vi "mul.vi"(11 "arguments":T1[](array[typedef])) -> (3 "Expression":T1)   [LabVIEW 2020]
uses:
  ExpressionType.ctl
  Expression.ctl
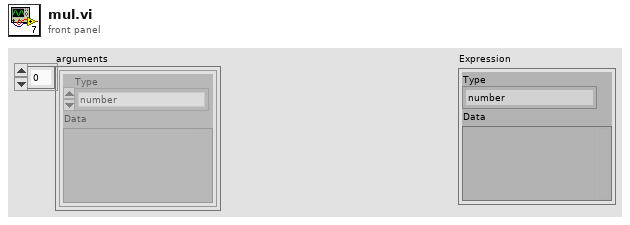
[diagram p1: front panel]
types:
  T1 = typedef "Expression.ctl" = cluster{"Type":T2, "Data":variant}
  T2 = typedef "ExpressionType.ctl" = enum16{"number", "string", "symbol", "primitive", "list", "closure", "macro", "nil", "error"}
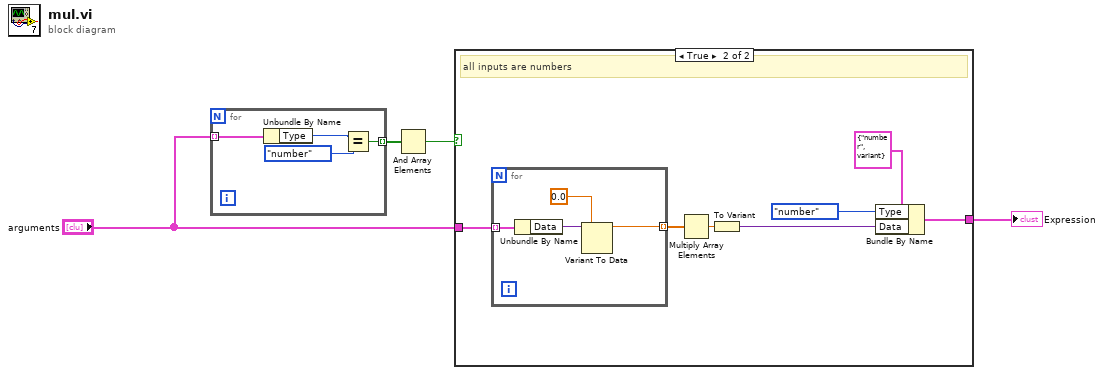
[diagram p0: block diagram]
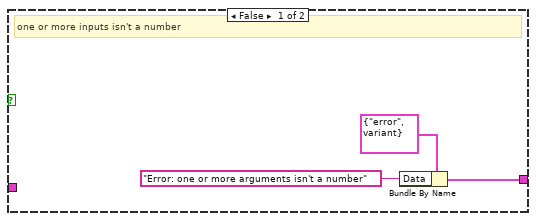
[diagram p2: hidden frame]
diagram:
  n1 = for {
    tunnel: "arguments" -> [w8] mode=indexing
    tunnel: [w5] -> w2 mode=indexing
    n2 = Unbundle By Name(w8) -> ("Type"=w7:T2)
    n3 = Equal?(x=w7, y=ExpressionType."number") -> (x = y?=w5:bool)
  }
  n4 = And Array Elements(Boolean array=w2) -> (logical AND=w1:bool)
  n5 = case shown="True" w1 {
    tunnel: [w10 w16] -> w4
    tunnel: "arguments" -> [_ w12]
    frame False {
      # "one or more inputs isn't a number"
      n6 = Bundle By Name(cluster=T1 {"Type"=enum."error", "Data"=variant} ("Expression 3"), "Data"="Error: one or more arguments isn't a number") -> (w10:T1)
    }
    frame True {
      # "all inputs are numbers"
      n7 = for {
        tunnel: w12 -> [w22] mode=indexing
        tunnel: [w19] -> w14 mode=indexing
        n8 = Unbundle By Name(w22) -> ("Data"=w21:variant)
        n9 = Variant To Data(type=0.0, Variant=w21) -> (data=w19:dbl)  [unwired: 1 in, 1 out]
      }
      n10 = Multiply Array Elements(1:w14) -> (0:w13:dbl)
      n11 = To Variant(anything=w13) -> (Variant=w15:variant)
      n12 = Bundle By Name(cluster=T1 {"Type"=enum."number", "Data"=variant} ("Expression 3"), "Type"=ExpressionType."number" ("ExpressionType"), "Data"=w15) -> (w16:T1)
    }
  }
  "Expression" <- w4
